vi "Drop Messages.vi"(8 "error in":errorcluster, 11 "log in":T1) -> (0 "error out":errorcluster, 2 "Current Msgs":string[](array[string]), 3 "log out":T1)   [LabVIEW 2014, in "System Log.lvclass"]
doc: "Drop all messages in the current message queue."
uses:
  System Log.lvclass
  <userlib>/_Session Fwk/Typedefs/Session Handle.ctl
  <userlib>/_Session Fwk/Session - Root.lvclass
  System Log.lvclass/System Log.ctl
  Accessors/Read Current Message.vi
  Accessors/Write Current Message.vi
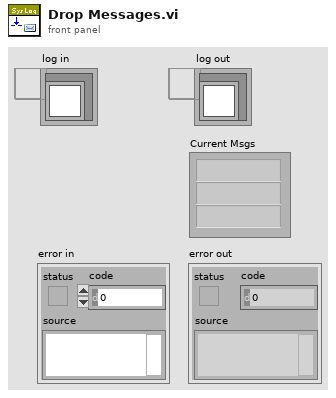
[diagram p1: front panel]
types:
  T1 = typedef "Session - Root.lvclass/Session Handle.ctl" = refnum<data-value>
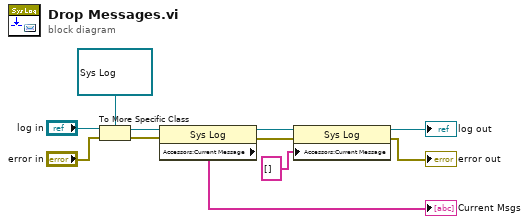
[diagram p0: block diagram]
diagram:
  n1 = To More Specific Class(target class=refnum<data-value> refnum ("log"), reference="log in", error in="error in") -> (specific class reference=w9:refnum<data-value>, error out=w2:errorcluster)
  n2 = property class="Sys Log"(reference=w9, error in=w2) -> (reference out=w8:refnum<data-value>, error out=w1:errorcluster, "Accessors:Current Message"=→"Current Msgs":string[])
  n3 = property class="Sys Log"(reference=w8, error in=w1, "Accessors:Current Message"=string[] [] ("Current Msgs")) -> (reference out=→"log out":refnum<data-value>, error out=→"error out":errorcluster)
